vi "R2 Time SBR Cycle.vi"(10 "Pump Status Array":bool[][](array[boolean])=[[TRUE, FALSE, TRUE, FALSE, FALSE], [TRUE, FALSE, FALSE, FALSE, TRUE], [FALSE, FALSE, FALSE, TRUE, FALSE], [FALSE, FALSE, FALSE, FALSE, FALSE], [FALSE, TRUE, FALSE, FALSE, FALSE], [FALSE, FALSE, FALSE, FALSE, FALSE]], 11 "Array":dbl[](array[numeric])) -> ()   [LabVIEW 2016]
uses:
  R2 Pump Manual Control.ctl
  R2Variables.lvlib
panel:
  in  "stop":bool
  out "Phase":dbl
  # "Call from Control.vi"
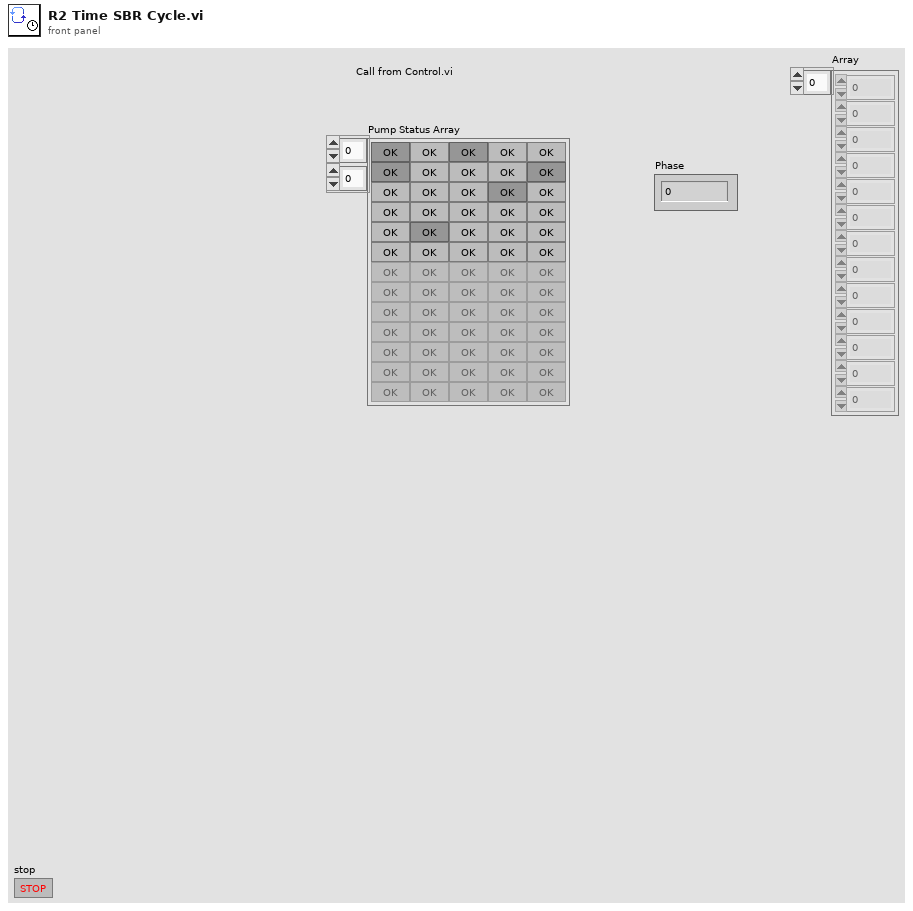
[diagram p1: front panel]
types:
  T1 = typedef "R2Variables.lvlib/R2 Pump Manual Control.ctl" = cluster{"Water Pump":bool, "Effluent Pump":bool, "Media Pump":bool, "Gas Pump":bool, "Air Release Valve":bool, "Floc Effluent Pump":bool, "Floc Return Pump":bool, "Floc Air Valve":bool}
  T2 = cluster{"Pump Status Array[0]":bool, "Pump Status Array[1]":bool, "Pump Status Array[2]":bool, "Pump Status Array[3]":bool, "Pump Status Array[4]":bool, "Pump Status Array[5]":bool, "Pump Status Array[6]":bool, "Pump Status Array[7]":bool, "Pump Status Array[8]":bool}
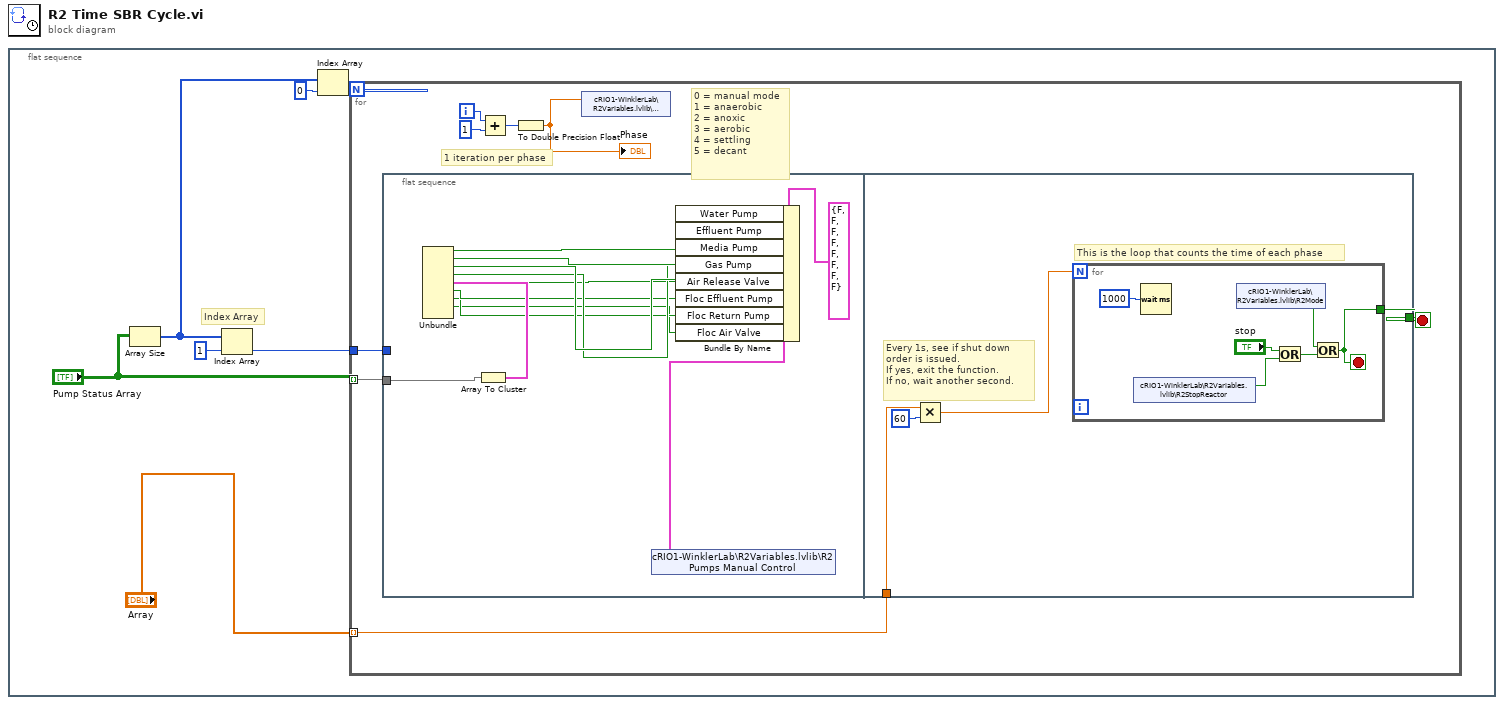
[diagram p0: block diagram]
diagram:
  n1 = flat-sequence {
    frame #0 {
      # "Index Array"
      n2 = Array Size(array="Pump Status Array") -> (size(s)=w5:i32[])
      n3 = Index Array(array=w5, index=1) -> (element=w6:i32)
      n4 = Index Array(array=w5, index=0) -> (element=w2:i32)
      n5 = for {
        N: w2 -> [_]
        tunnel: "Array" -> [w13] mode=indexing
        tunnel: w6 -> [w15]
        tunnel: "Pump Status Array" -> [w14] mode=indexing
        i -> [w12]
        stop <- w8 stop-if-true
        # "0 = manual mode\n1 = anaerobic\n2 = anoxic\n3 = aerobic\n4 = settling\n5 = decant"
        # "1 iteration per phase"
        n6 = flat-sequence {
          tunnel: w15 -> [_]
          tunnel: w14 -> [w27]
          tunnel: w13 -> [w30]
          tunnel: [w29] -> w8
          frame #0 {
            n7 = Array To Cluster(array=w27) -> (cluster=w26:T2)
            n8 = Unbundle(w26) -> ("Pump Status Array[0]"=w24:bool, "Pump Status Array[1]"=w23:bool, "Pump Status Array[2]"=w22:bool, "Pump Status Array[3]"=w21:bool, "Pump Status Array[4]"=w20:bool, "Pump Status Array[5]"=w18:bool, "Pump Status Array[6]"=w17:bool, "Pump Status Array[7]"=w16:bool)  [unwired: 1 out]
            n9 = Bundle By Name(cluster=T1 {"Water Pump"=FALSE, "Effluent Pump"=FALSE, "Media Pump"=FALSE, "Gas Pump"=FALSE, "Air Release Valve"=FALSE, "Floc Effluent Pump"=FALSE, "Floc Return Pump"=FALSE, "Floc Air Valve"=FALSE} ("Reactor 2 SBR Control"), "Water Pump"=w24, "Effluent Pump"=w23, "Media Pump"=w22, "Gas Pump"=w21, "Air Release Valve"=w20, "Floc Effluent Pump"=w18, "Floc Return Pump"=w17, "Floc Air Valve"=w16) -> (w19:T1)
            n10 = shared-variable "cRIO1-WinklerLab\\R2Variables.lvlib\\R2 Pumps Manual Control"(w19) -> ()  [unwired: 1 in, 1 out]
          }
          frame #1 {
            # "This is the loop that counts the time of each phase"
            # "Every 1s, see if shut down order is issued.\nIf yes, exit the function.\nIf no, wait another second."
            n11 = Multiply(x=w30, y=u32 60) -> (x*y=w28:dbl)
            n12 = for {
              N: w28 -> [_]
              tunnel: [w33] -> w29
              stop <- w33 stop-if-true
              n13 = shared-variable "cRIO1-WinklerLab\\R2Variables.lvlib\\R2StopReactor"() -> (w32:bool)  [unwired: 1 in, 1 out]
              n14 = Wait (ms)(milliseconds to wait=u32 1000) -> ()  [unwired: 1 out]
              n15 = shared-variable "cRIO1-WinklerLab\\R2Variables.lvlib\\R2Mode"() -> (w34:bool)  [unwired: 1 in, 1 out]
              n16 = Or(x="stop", y=w32) -> (x .or. y?=w35:bool)
              n17 = Or(x=w34, y=w35) -> (x .or. y?=w33:bool)
            }
          }
        }
        n18 = Add(x=w12, y=1) -> (x+y=w10:i32)
        n19 = To Double Precision Float(number=w10) -> (double precision float=w9:dbl)
        "Phase" <- w9
        n20 = shared-variable "cRIO1-WinklerLab\\R2Variables.lvlib\\R2Phase"(w9) -> ()  [unwired: 1 in, 1 out]
      }
    }
  }
